vi "Core.vi"(8 "error in (no error)":errorcluster, 10 "Actor in":refnum<class "Actor.lvclass">, 11 "Data Tracker Msg in":refnum<class "Data Tracker Msg.lvclass">) -> (0 "error out":errorcluster, 1 "Data":refnum<class "Data.lvclass">, 2 "Actor out":refnum<class "Actor.lvclass">, 3 "Data Tracker Msg out":refnum<class "Data Tracker Msg.lvclass">)   [LabVIEW 2020, in "Data Tracker.lvlib" / "Data Tracker Msg.lvclass"]
doc: "Core of the Reponse Msg. Put the active code here.\n\nThis implementation either Start, Ends or Aborts tracking as specified by the Data Tracker Msg."
uses:
  Data Tracker Msg.lvclass
  PPL/HDH.Data.Generic.lvlibp/Data.lvclass
  PPL/HDH.Actor Framework.Core.Actor.lvlibp/1abvi3w/vi.lib/ActorFramework/Actor/Actor.lvclass
  Data Tracker/Data Tracker.lvclass
  C:/Current projects/WS/PPL/HDH.Actor Framework.Core.Actor.lvlibp/1abvi3w/vi.lib/ActorFramework/Actor/Actor.lvclass
  Data Tracker Msg.lvclass/Data Tracker Msg.ctl
  Data Tracker/Data/Tracker Data.lvclass/Tracker Data.ctl
  Data Tracker/Data/Tracker Data.lvclass
  C:/Current projects/WS/PPL/HDH.Data.Generic.lvlibp/Data.lvclass
  PPL/HDH.Actor Framework.Core.Publisher.lvlibp/Messages/Timed Msg/Data/Timed Data/Timed Data.lvclass
  PPL/HDH.Actor Framework.Core.Publisher.lvlibp/Messages/Timed Msg/Timed Msg.lvclass
  C:/Current projects/WS/PPL/HDH.Actor Framework.Core.Publisher.lvlibp/Messages/Timed Msg/Data/Timed Data/Timed Data.lvclass
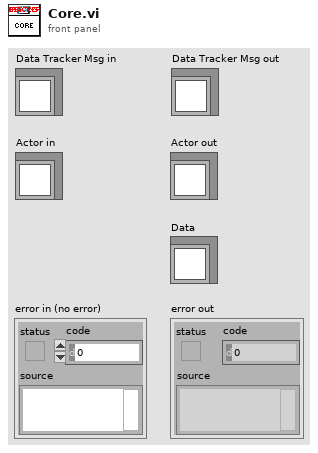
[diagram p1: front panel]
types:
  T1 = typedef "Data Tracker.lvlib/Ctl_Action.ctl" = enum16{"Start Tracking", "End Tracking", "Abort Tracking"}
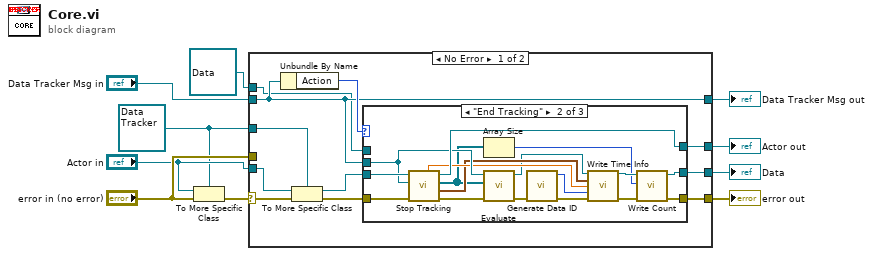
[diagram p0: block diagram]
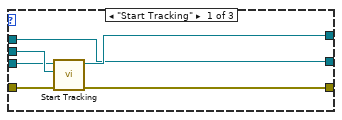
[diagram p2: hidden frame]
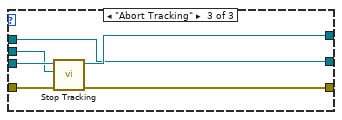
[diagram p3: hidden frame]
diagram:
  w5 = refnum<class "Data Tracker.lvclass"> refnum ("Data Tracker.lvlib:Data Tracker.lvclass")
  n1 = To More Specific Class(target class=w5, reference="Actor in", error in="error in (no error)") -> (error out=w10:errorcluster)  [unwired: 1 out]
  n2 = case shown="No Error" w10 {
    selector: w10 -> [w21 _]
    tunnel: [w14 w54] -> w9
    tunnel: "error in (no error)" -> [_ w54]
    tunnel: [w16 w53] -> w7
    tunnel: "Actor in" -> [w20 w53]
    tunnel: w5 -> [w19 _]
    tunnel: [w13 w52] -> w4
    tunnel: "Data Tracker Msg in" -> [w13 w52]
    tunnel: [w12 w51] -> w2
    tunnel: refnum<class "Data.lvclass"> refnum ("Data") -> [w11 w51]
    frame No Error {
      n3 = Unbundle By Name(w13) -> ("Action"=w18:T1)
      n4 = To More Specific Class(target class=w19, reference=w20, error in=w21) -> (specific class reference=w17:refnum<class "Data Tracker.lvclass">, error out=w15:errorcluster)
      n5 = case shown="\"End Tracking\"" w18 {
        tunnel: w13 -> [w27 w40 w48]
        tunnel: w17 -> [w26 w44 w50]
        tunnel: [w25 w43 w49] -> w16
        tunnel: w15 -> [w24 w42 w47]
        tunnel: [w23 w32 w46] -> w14
        tunnel: [w22 w30 w45] -> w12
        tunnel: w11 -> [w22 _ w45]
        frame "Start Tracking" {
          n6 = call "Start Tracking.vi"("error in (no error)"=w24, "Tracker Type"=w27, "Data Tracker in"=w26) -> ("error out"=w23:errorcluster, "Data Tracker out"=w25:refnum<class "Data Tracker.lvclass">)  [unwired: 7 in]
        }
        frame "End Tracking" {
          n7 = call "Stop Tracking.vi"("error in (no error)"=w42, "Tracker Type"=w40, "Data Tracker in"=w44) -> ("error out"=w41:errorcluster, "Start Time"=w35:timestamp, "Data"=w29:refnum<class "Data.lvclass">[], "Data Tracker out"=w43:refnum<class "Data Tracker.lvclass">, "Duration(s)"=w36:dbl)  [unwired: 4 in]
          n8 = Array Size(array=w29) -> (size(s)=w28:i32)
          n9 = call-dynamic "Evaluate.vi"("error in (no error)"=w41, "Data"=w29, "Data Tracker Msg in"=w40) -> ("error out"=w38:errorcluster, "Tracker Data"=w33:refnum<class "Tracker Data.lvclass">)  [unwired: 7 in]
          n10 = call "Generate Data ID.vi"("error in (no error)"=w38) -> ("error out"=w37:errorcluster, "Data ID"=w39:u32)  [unwired: 9 in]
          n11 = call "Write Time Info.vi"("Request Data in"=w33, "Start TIme"=w35, "Duration(s)"=w36, "Data ID"=w39, "error in (no error)"=w37) -> ("Request Data out"=w31:refnum<class "Tracker Data.lvclass">, "error out"=w34:errorcluster)  [unwired: 9 in]
          n12 = call "Write Count.vi"("error in (no error)"=w34, "Data Count"=w28, "Tracker Data in"=w31) -> ("error out"=w32:errorcluster, "Tracker Data out"=w30:refnum<class "Tracker Data.lvclass">)  [unwired: 7 in]
        }
        frame "Abort Tracking" {
          n13 = call "Stop Tracking.vi"("error in (no error)"=w47, "Tracker Type"=w48, "Data Tracker in"=w50) -> ("error out"=w46:errorcluster, "Data Tracker out"=w49:refnum<class "Data Tracker.lvclass">)  [unwired: 4 in, 3 out]
        }
      }
    }
    frame Error {
    }
  }
  "error out" <- w9
  "Actor out" <- w7
  "Data" <- w2
  "Data Tracker Msg out" <- w4
